vi "SVT UFF58 Write Record 5.vi"(0 "function refnum":refnum<k20>, 5 "record 5":string, 11 "error in (no error)":errorcluster) -> (4 "dup function refnum":refnum<k20>, 15 "error out":errorcluster)   [LabVIEW 2017, in "SoundVib_UFF58.lvlib"]
doc: "Writes the values of the fields in record 5 of the UFF58 (universal file format) file."
uses:
  <vilib>/addons/Sound and Vibration/svt_UFF58/SoundVib_UFF58.lvlib
  <vilib>/Platform/storage/Storage.llb/Set Property (String).vi
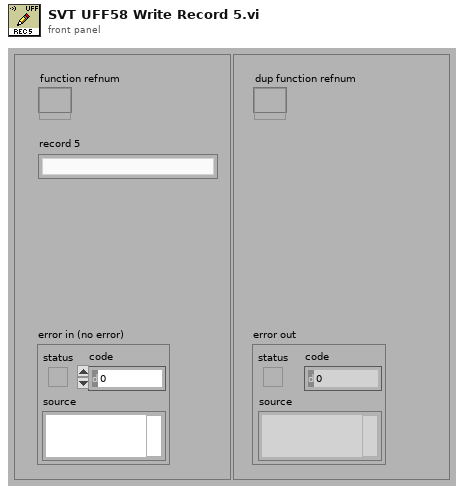
[diagram p1: front panel]
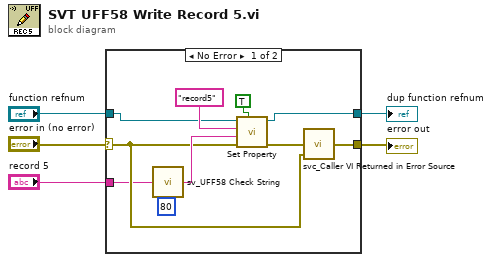
[diagram p0: block diagram]
diagram:
  n1 = case shown="No Error" "error in (no error)" {
    selector: "error in (no error)" -> [w10 w16]
    tunnel: "function refnum" -> [w14 w17]
    tunnel: [w6 w17] -> w2
    tunnel: [w11 w16] -> w5
    tunnel: "record 5" -> [w8 _]
    frame No Error {
      n2 = call <vilib>:"sv_UFF58 Check String.vi"("field value"=w8, "field length"=80 ("length (rest)")) -> ("output string"=w13:string)  [unwired: 12 in, 1 out]
      n3 = call-poly <vilib>:"Set Property.vi"("Create if not found (no:F)"=TRUE, "error in (no error)"=w10, "Value"=w13, "Property name"="record5", "storage refnum"=w14) -> ("error out"=w7:errorcluster, "storage refnum out"=w6:refnum<k20>)  [unwired: 5 in]
      n4 = call <vilib>:"svc_Caller VI Returned in Error Source.vi"("warning input to caller"=w10, "error in (no error)"=w7) -> ("error out"=w11:errorcluster)  [unwired: 3 in]
    }
    frame Error {
    }
  }
  "error out" <- w5
  "dup function refnum" <- w2
